vi "Read summaryState.vi"(11 "ComponentData in":refnum<class "ComponentData.lvclass">) -> (2 "ComponentState.lvclass":refnum<class "ComponentState.lvclass">, 3 "ComponentData out":refnum<class "ComponentData.lvclass">)   [LabVIEW 2013, in "ComponentData.lvlib" / "ComponentData.lvclass"]
uses:
  <userlib>/Common/Component/common_application/RT/ComponentData/ComponentData/ComponentData.lvclass
  <userlib>/Common/Component/common_application/RT/ComponentData/ComponentState/ComponentState/ComponentState.lvclass
  <userlib>/Common/Component/common_application/RT/ComponentData/ComponentData/ComponentData.lvclass/ComponentData.ctl
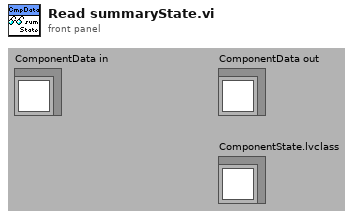
[diagram p1: front panel]
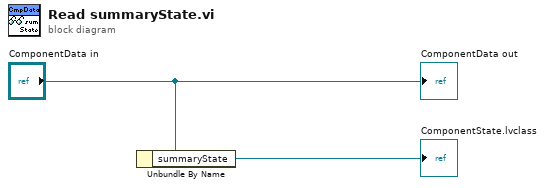
[diagram p0: block diagram]
diagram:
  n1 = Unbundle By Name("ComponentData in") -> ("summaryState"=→"ComponentState.lvclass":refnum<class "ComponentState.lvclass">)
  "ComponentData out" <- "ComponentData in"
